vi "Test.vi"   [LabVIEW 2018, in "Scripts.lvlib"]
uses:
  Scripts.lvlib
  tests/Tests.lvlib
  <vilib>/addons/_JKI Toolkits/Caraya/classes/Test/Test.lvclass
panel:
  # "Overview: Executes all of the tests for this project\nRequirements: LabVIEW, Caraya Unit Testing Framework\nInstructions: Run this VI.\n\nThis VI will run all of the tests as defined using the Caraya unit testing framework."
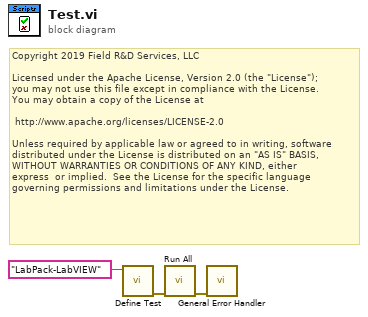
[diagram p0: block diagram]
diagram:
  # "Copyright 2019 Field R&D Services, LLC\n\nLicensed under the Apache License, Version 2.0 (the \"License\");\nyou may not use this file except in compliance with the License.\nYou may obtain a copy of the License at\n\n\thttp://www.apache.org/licenses/LICENSE-2.0\n\nUnless required by applicable law or agreed to in writing, software\ndistributed under the License is distributed on an \"AS IS\" BASIS,\nWITHOUT WARRANTIES OR CONDITIONS OF ANY KIND, either \nexpress  or implied.  See the License for the specific language \ngoverning permissions and limitations under the License."
  n1 = call <vilib>:"Define Test.vi"("Label (VI Title)"="LabPack-LabVIEW") -> ("error out"=w3:errorcluster)  [unwired: 10 in]
  n2 = call "Run All.vi"("Error In"=w3) -> ("Error Out"=w1:errorcluster)  [unwired: 10 in]
  n3 = call <vilib>:"General Error Handler.vi"("error in (no error)"=w1) -> ()  [unwired: 10 in, 5 out]
